vi "Write.vi"(8 "error in":errorcluster, 9 "File Name":string=" Test.txt", 11 "text":string) -> (0 "error out":errorcluster)   [LabVIEW 2020]
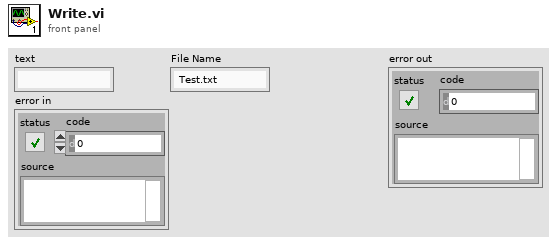
[diagram p1: front panel]
types:
  T1 = enum16{"open", "replace", "create", "open or create", "replace or create", "replace or create with confirmation"}
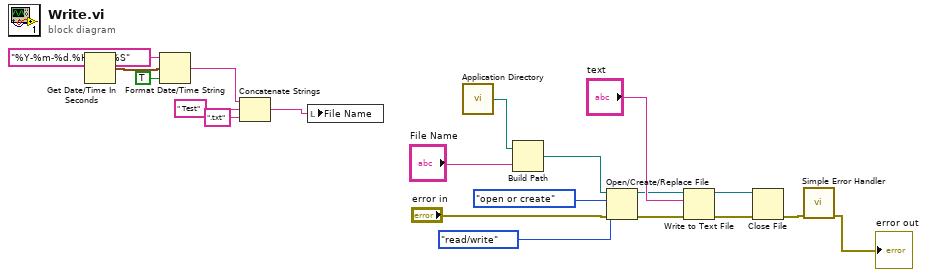
[diagram p0: block diagram]
diagram:
  n1 = Get Date/Time In Seconds() -> (seconds since 1Jan1904=w7:timestamp)
  n2 = Format Date/Time String(time format string (%c)="%Y-%m-%d.%H-%M-%S", seconds (now)=w7, UTC format=TRUE) -> (date/time string=w5:string)
  n3 = Concatenate Strings(w5, " Test" ("string"), ".txt" ("string")) -> (w1:string)
  n4 = local write "File Name"(w1) -> ()
  n5 = call <vilib>:"Application Directory.vi"() -> ("Application Directory"=w9:path)
  n6 = Build Path(base path=w9, name or relative path="File Name") -> (appended path=w13:path)
  n7 = Open/Create/Replace File(file path (use dialog)=w13, error in="error in", operation (0:open)=T1."open or create", access (0:read/write)=enum16{"read/write", "read-only", "write-only"}."read/write") -> (refnum out=w12:refnum<file>, error out=w17:errorcluster)  [unwired: 2 in, 1 out]
  n8 = Write to Text File(file (use dialog)=w12, text="text", error in=w17) -> (refnum out=w16:refnum<file>, error out=w15:errorcluster)  [unwired: 1 in, 1 out]
  n9 = Close File(refnum=w16, error in=w15) -> (error out=w11:errorcluster)  [unwired: 1 out]
  n10 = call <vilib>:"Simple Error Handler.vi"("error in (no error)"=w11) -> ("error out"=→"error out":errorcluster)  [unwired: 4 in, 4 out]
